vi "GetThePosition.vi"(5 "Property Array":string[](array[string]), 7 "Physical Channel Array":string[](array[string]), 8 "error IO":errorcluster, 10 "Position Index In":T1, 11 "Data in":T2) -> (0 "error out":errorcluster, 3 "Position Index Out":T1)   [LabVIEW 2018]
uses:
  Ctrl/Data.ctl
  Ctrl/Caps.ctl
  Ctrl/Property.ctl
  Ctrl/PhysicalChannel.ctl
  Ctrl/Register.ctl
  Ctrl/Bitfield.ctl
  Ctrl/Scale.ctl
  Ctrl/ScaleType.ctl
  Ctrl/Enum.ctl
  Ctrl/EnumValue.ctl
  e12b2da5-091d-4e13-bb1e-f6d335301894.vi
  707d1d17-c49e-4b72-b4e4-1888d512a412.vi
  cf412191-4968-46c8-a1c6-7b874dfe2e2c.vi
  <vilib>/JDP Science/JSONtext/String Subset.vi
  <vilib>/JDP Science/JSONtext/Parsing/Parse Full Path or Item Name.vi
  <vilib>/JDP Science/JSONtext/Offset/Find Item Locations by Path.vi
  <vilib>/JDP Science/JSONtext/JSON text to Variant.vi
  <vilib>/JDP Science/JSONtext/JSONtext.lvlib
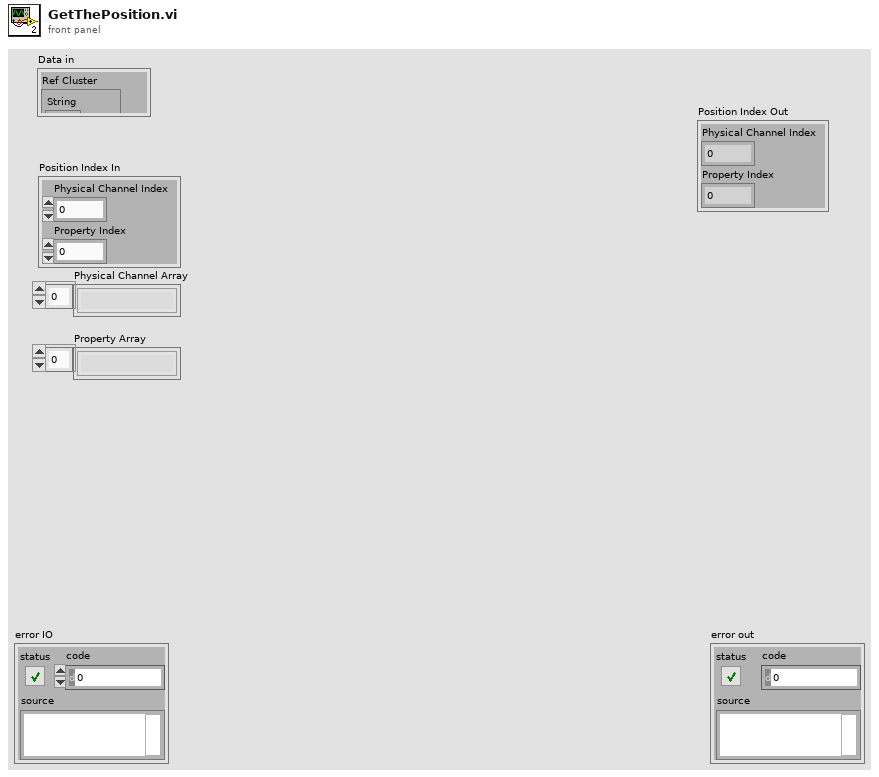
[diagram p1: front panel]
types:
  T1 = cluster{"Physical Channel Index":i32, "Property Index":i32}
  T2 = typedef "Data.ctl" = cluster{"Ref Cluster":cluster{"String":refnum<vi>, "U8":refnum<vi>, "I8":refnum<vi>, "U32":refnum<vi>, "I32":refnum<vi>, "U64":refnum<vi>, "I64":refnum<vi>, "Ring":refnum<vi>, "DBL":refnum<vi>, "Add":refnum<vi>, "Remove":refnum<vi>, "Property tree":refnum<vi>, "confirm":refnum<vi>}, "JSON Text":string, "Original JSON Text":string, "Caps":T3, "SLSC Output Tree":cluster{"Left Cell String":string, "Child Text":string[], "Child Tag":string, "Item Indent":i32, "Child Only?":bool, "Glyph Index":i32, "offline value":variant}[], "Ref Index and Control Type":cluster{"index":i32, "Datatype":string}, "Selected Type and name":cluster{"Selected Type":enum16{"Property", "Physical Channel", "Other"}, "Selected Property Name":string}, "Update whole Tree?":bool}
  T3 = typedef "Caps.ctl" = cluster{"properties":T4[], "physical channels":T5[], "registers":T6[], "scales":T8[], "enums":T10[], "productName":string}
  T4 = typedef "Property.ctl" = cluster{"name":string, "bitfield":string, "value":variant, "dataType":string, "min":variant, "max":variant, "scale":string, "access":string}
  T5 = typedef "PhysicalChannel.ctl" = cluster{"name":string, "properties":T4[]}
  T6 = typedef "Register.ctl" = cluster{"name":string, "address":i32, "size":i32, "bitfields":T7[], "initialValue":variant, "connectedProperties":string[]}
  T7 = typedef "Bitfield.ctl" = cluster{"name":string, "offset":i32, "size":i32, "signed":bool}
  T8 = typedef "Scale.ctl" = cluster{"name":string, "type":T9, "params":variant}
  T9 = typedef "ScaleType.ctl" = enum16{"NoScale", "Table", "Polynomial", "Linear"}
  T10 = typedef "Enum.ctl" = cluster{"name":string, "values":T11[]}
  T11 = typedef "EnumValue.ctl" = cluster{"name":string, "value":i32}
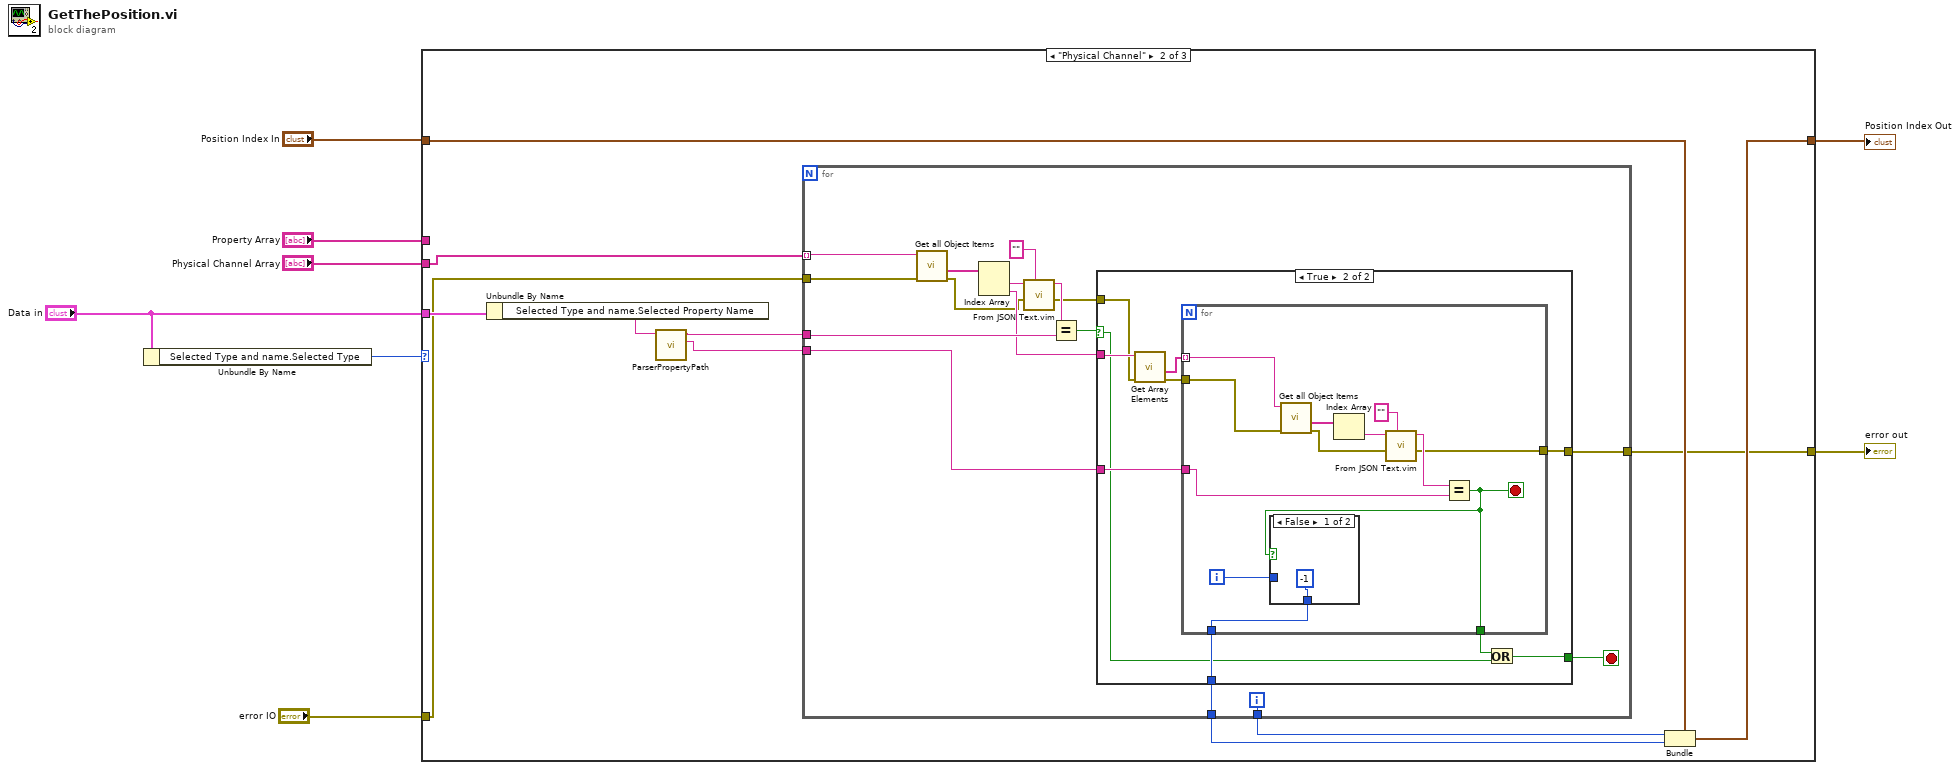
[diagram p0: block diagram]
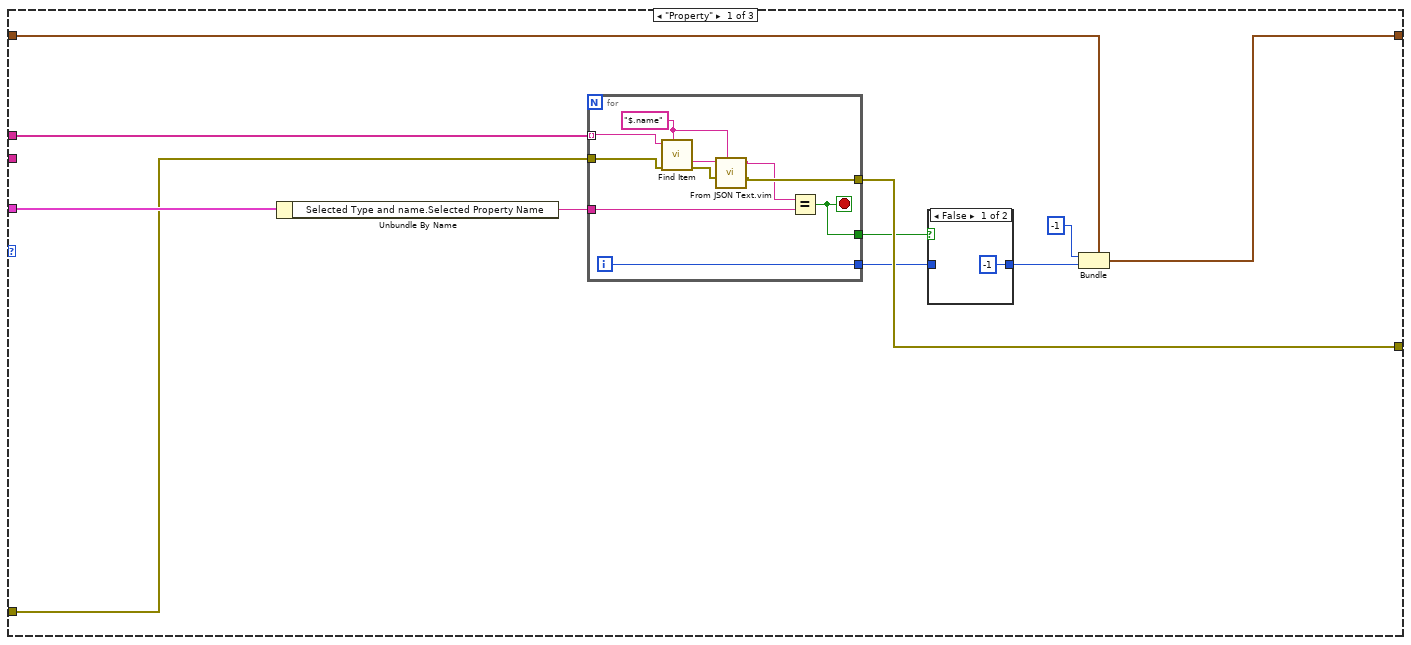
[diagram p2: hidden frame]
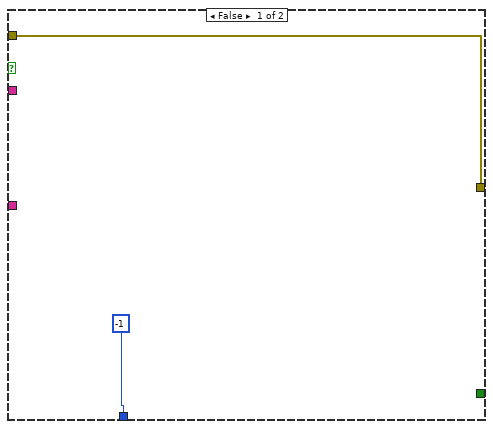
[diagram p4: hidden frame]
diagram:
  n1 = Unbundle By Name("Data in") -> ("Selected Type and name.Selected Type"=w1:enum16{"Property", "Physical Channel", "Other"})
  n2 = case shown="\"Physical Channel\"" w1 {
    tunnel: "Data in" -> [w17 w41 _]
    tunnel: "error IO" -> [w13 w36 w85]
    tunnel: "Physical Channel Array" -> [_ w42 _]
    tunnel: "Position Index In" -> [w16 w40 w86]
    tunnel: [w14 w37 w86] -> w6
    tunnel: "Property Array" -> [w18 _ _]
    tunnel: [w12 w35 w85] -> w5
    frame "Property" {
      n3 = Unbundle By Name(w17) -> ("Selected Type and name.Selected Property Name"=w19:string)
      n4 = for {
        tunnel: w18 -> [w27] mode=indexing
        tunnel: w19 -> [w31]
        tunnel: [w30] -> w11
        tunnel: w13 -> [w26]
        tunnel: [w24] -> w12
        tunnel: [w22] -> w10
        i -> [w30]
        stop <- w22 stop-if-true
        w28 = "$.name" ("$Path or Item Name")
        n5 = call <vilib>:"Find Item.vi"("$Path or Item Name"=w28, "error in (no error)"=w26, "JSON"=w27) -> ("error out"=w25:errorcluster, "<JSON>"=w29:string)  [unwired: 5 in, 2 out]
        n6 = call "From JSON Text.vim"("Data Type and Default Value"=w28, "error in (no error)"=w25, "JSON"=w29) -> ("error out"=w24:errorcluster, "Data out"=w23:string)  [unwired: 7 in]
        n7 = Equal?(x=w23, y=w31) -> (x = y?=w22:bool)
      }
      n8 = case shown="False" w10 {
        tunnel: w11 -> [_ w21]
        tunnel: [-1 w21] -> w9
        frame False {
        }
        frame True {
        }
      }
      n9 = Bundle(cluster=w16, "Physical Channel Index"=-1, "Property Index"=w9) -> (w14:T1)
    }
    frame "Physical Channel" {
      n10 = Unbundle By Name(w41) -> ("Selected Type and name.Selected Property Name"=w32:string)
      n11 = call "ParserPropertyPath.vi"("property"=w32) -> ("name"=w33:string, "pyhsical channel"=w34:string)  [unwired: 7 in]
      n12 = for {
        tunnel: w42 -> [w58] mode=indexing
        tunnel: w33 -> [w50]
        tunnel: w34 -> [w53]
        tunnel: [w48] -> w39
        tunnel: [w47] -> w38
        tunnel: w36 -> [w46]
        tunnel: [w43] -> w35
        i -> [w48]
        stop <- w49 stop-if-true
        n13 = call <vilib>:"Get all Object Items.vi"("error in (no error)"=w46, "JSON"=w58) -> ("error out"=w45:errorcluster, "<JSON>"=w57:string[])  [unwired: 6 in, 2 out]
        n14 = Index Array(array=w57) -> (element #1=w56:string, element #2=w51:string)  [unwired: 2 in]
        n15 = call "From JSON Text.vim"("Data Type and Default Value"="", "error in (no error)"=w45, "JSON"=w56) -> ("error out"=w44:errorcluster, "Data out"=w55:string)  [unwired: 7 in]
        n16 = Equal?(x=w55, y=w53) -> (x = y?=w52:bool)
        n17 = case shown="True" w52 {
          selector: w52 -> [_ w61]
          tunnel: w51 -> [_ w70]
          tunnel: w50 -> [_ w68]
          tunnel: [_ w62] -> w49
          tunnel: [-1 w66] -> w47
          tunnel: w44 -> [w60 w65]
          tunnel: [w60 w63] -> w43
          frame False {
          }
          frame True {
            n18 = call <vilib>:"Get Array Elements.vi"("error in (no error)"=w65, "JSON"=w70) -> ("error out"=w64:errorcluster, "<JSON>"=w69:string[])  [unwired: 7 in, 1 out]
            n19 = for {
              tunnel: w69 -> [w82] mode=indexing
              tunnel: w68 -> [w77]
              tunnel: [w73] -> w67
              tunnel: [w71] -> w66
              tunnel: w64 -> [w76]
              tunnel: [w74] -> w63
              i -> [w72]
              stop <- w73 stop-if-true
              n20 = call <vilib>:"Get all Object Items.vi"("error in (no error)"=w76, "JSON"=w82) -> ("error out"=w75:errorcluster, "<JSON>"=w81:string[])  [unwired: 6 in, 2 out]
              n21 = Index Array(array=w81) -> (element=w80:string)  [unwired: 1 in]
              n22 = call "From JSON Text.vim"("Data Type and Default Value"="", "error in (no error)"=w75, "JSON"=w80) -> ("error out"=w74:errorcluster, "Data out"=w78:string)  [unwired: 7 in]
              n23 = Equal?(x=w78, y=w77) -> (x = y?=w73:bool)
              n24 = case shown="False" w73 {
                tunnel: w72 -> [_ w84]
                tunnel: [-1 w84] -> w71
                frame False {
                }
                frame True {
                }
              }
            }
            n25 = Or(x=w67, y=w61) -> (x .or. y?=w62:bool)
          }
        }
      }
      n26 = Bundle(cluster=w40, "Physical Channel Index"=w39, "Property Index"=w38) -> (w37:T1)
    }
    frame "Other", Default {
    }
  }
  "Position Index Out" <- w6
  "error out" <- w5
